vi "Execute VI Analyzer Tests.vi"(8 "error in":errorcluster, 9 "File Name":string, 10 "File List":path[](array[path]), 11 "Peer Review in":refnum<class "Peer Review.lvclass">) -> (0 "error out":errorcluster, 3 "Peer Review out":refnum<class "Peer Review.lvclass">)   [LabVIEW 2020, in "Peer Review.lvclass"]
uses:
  Peer Review.lvclass
  Peer Review.lvclass/Peer Review.ctl
  <vilib>/addons/analyzer/NI_VIAnalyzerTKVIs.lvlib
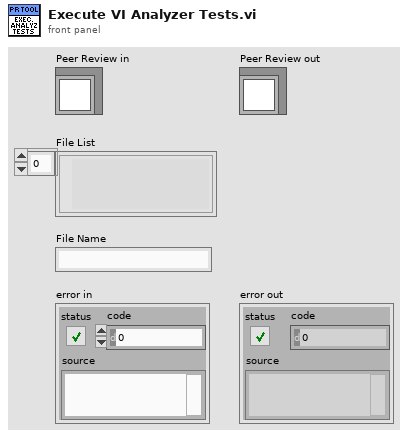
[diagram p1: front panel]
types:
  T1 = typedef "Peer Review.lvclass/File Info.ctl" = cluster{"File ID":i32, "Commit ID":i32, "Reviewed Hash":string, "Relative Path":string, "File Path":path, "File Checksum":string, "State":T2, "FP Changes":i32, "BD Changes":i32, "FP Bounds Error":dbl, "BD Bounds Error":dbl, "Lines Added":i32, "Lines Removed":i32, "Analysis Passes":i32, "Analysis Fails":i32, "Attribute Changes":i32, "Reentrancy State":string, "Cyclomatic Complexity":i32, "Node Count":i32, "Revision Number":u32, "LabVIEW Version":string, "Description":string, "Master Path":path, "Master Checksum":string, "VI Type":T3, "LabVIEW File":bool, "Review Complete":bool, "File Ref":refnum<vi>}
  T2 = typedef "Peer Review.lvclass/File State.ctl" = enum16{"Interrogation Needed", "Modified", "Deleted", "Added", "Matches Previous", "No Changes", "Moved"}
  T3 = typedef "Peer Review.lvclass/VI Type.ctl" = enum32{"invalid VI type", "Standard VI", "Control VI", "Global VI", "Polymorphic VI", "Configuration VI", "SubSystem", "Facade VI", "Method VI", "Statechart Diagram VI"}
  T4 = typedef "VIAnAPI Ref.ctl" = refnum<k1>
  T5 = typedef "VIAnCtl Results.ctl" = cluster{"Test Name":string, "Results Data":T6[], "Status":T7, "Exceed Max Fails?":bool}
  T6 = typedef "VIAnCtl ResultsData (index).ctl" = cluster{"Result Message":string, "Ref Index":i32}
  T7 = typedef "VIAnCtl ResultStatus.ctl" = enum16{"Pass", "Fail", "Skipped", "VI not loadable", "Test not loadable", "Test not runnable", "Test error out"}
  T8 = typedef "VIAnRes Parsed Results Data (by VI).ctl" = cluster{"VI Path":path, "Pass":cluster{"row":i32, "column":i32}[], "Fail":cluster{"row":i32, "column":i32}[], "Skipped":cluster{"row":i32, "column":i32}[], "VI not loadable":cluster{"row":i32, "column":i32}[], "Test not loadable":cluster{"row":i32, "column":i32}[], "Test not runnable":cluster{"row":i32, "column":i32}[], "Test error out":cluster{"row":i32, "column":i32}[]}
  T9 = typedef "VIAnRes Parsed Results Data (by Test).ctl" = cluster{"Test Name":string, "Pass":cluster{"VI Path":path, "index":cluster{"row":i32, "column":i32}}[], "Fail":cluster{"VI Path":path, "index":cluster{"row":i32, "column":i32}}[], "Skipped":cluster{"VI Path":path, "index":cluster{"row":i32, "column":i32}}[]}
  T10 = typedef "VIAnCtl Test Config Data.ctl" = cluster{"Test Name":string, "Config Ref":refnum<vi>, "Ref Valid?":bool, "Test Ranking":T11, "Max Failures":u32, "Test Path":path, "Control Values":T12[], "Selected?":bool}
  T11 = typedef "VIAnCtl TestRanking.ctl" = u16
  T12 = typedef "VIAnCtl Config Control Value.ctl" = cluster{"Control Name":string, "Control Value":variant}
  T13 = cluster{"Raw Results":T5[][], "Parsed Results Data (by VI)":T8[], "Parsed Results Data (by Test)":T9[], "Summary Statistics":cluster{"Passed Tests":i32, "Failed Tests":i32, "Skipped Tests":i32, "VIs not loadable":i32, "Tests not loadable":i32, "Tests not runnable":i32, "Test error out":i32, "Start Time":u32, "Total Time (s)":dbl}, "Test Config Data":T10[]}
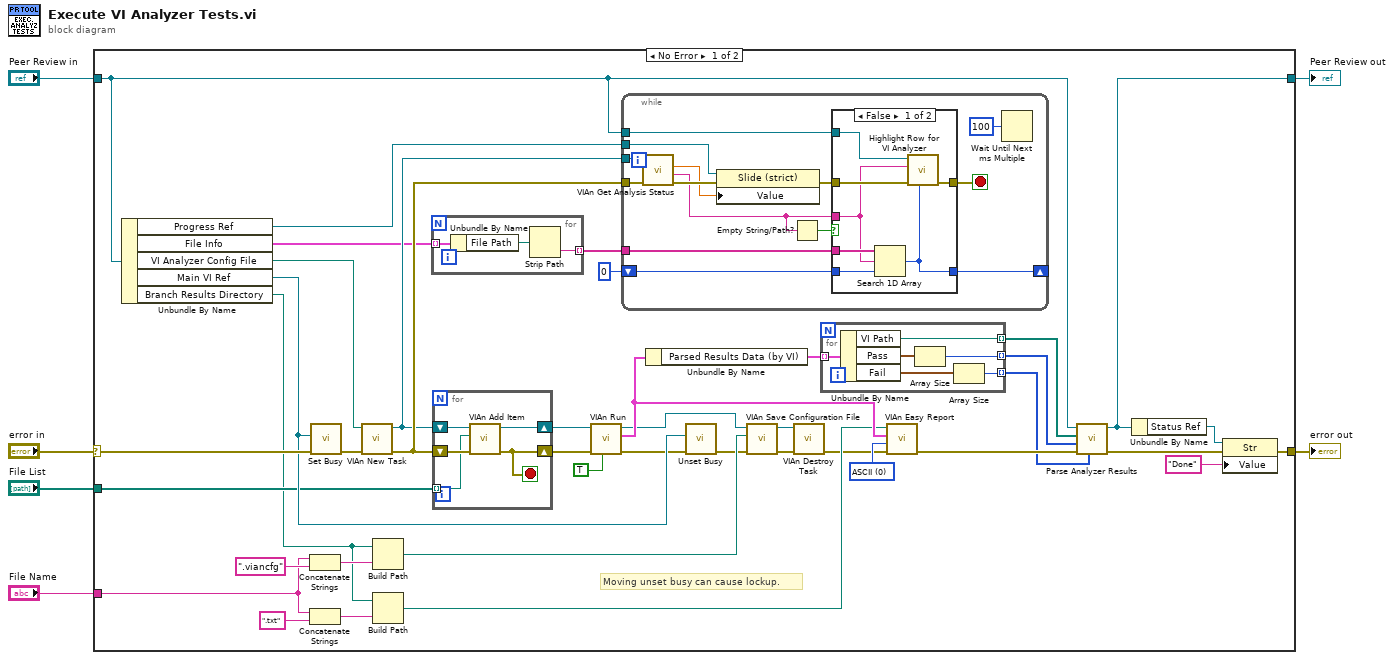
[diagram p0: block diagram]
diagram:
  n1 = case shown="No Error" "error in" {
    selector: "error in" -> [w33 w86]
    tunnel: [w13 w86] -> w6
    tunnel: "Peer Review in" -> [w15 w85]
    tunnel: [w14 w85] -> w4
    tunnel: "File Name" -> [w11 _]
    tunnel: "File List" -> [w26 _]
    frame No Error {
      w22 = u16 0 items=["ASCII", "HTML", "RSL File"] ("Report Save Type (ASCII)")
      # "Moving unset busy can cause lockup."
      n2 = Unbundle By Name(w15) -> ("Progress Ref"=w7:refnum<vi>, "File Info"=w10:T1[], "VI Analyzer Config File"=w47:path, "Main VI Ref"=w31:refnum<vi>, "Branch Results Directory"=w16:path)
      n3 = Concatenate Strings(w11, ".viancfg") -> (w35:string)
      n4 = Concatenate Strings(w11, ".txt") -> (w36:string)
      n5 = call <vilib>:"Set Busy.vi"("error in (no error)"=w33, "VI reference (current VI)"=w31) -> ("error out"=w18:errorcluster)  [unwired: 8 in, 1 out]
      n6 = call <vilib>:"VIAn New Task.vi"("error in (no error)"=w18, "Path to Configuration File"=w47) -> ("error out"=w20:errorcluster, "VI Analyzer Task"=w19:T4)  [unwired: 1 in, 7 out]
      n7 = Build Path(base path=w16, name or relative path=w35) -> (appended path=w37:path)
      n8 = Build Path(base path=w16, name or relative path=w36) -> (appended path=w38:path)
      n9 = for {
        tunnel: w10 -> [w50] mode=indexing
        tunnel: [w48] -> w8 mode=indexing
        n10 = Unbundle By Name(w50) -> ("File Path"=w49:path)
        n11 = Strip Path(path=w49) -> (name=w48:string)  [unwired: 1 out]
      }
      n12 = for {
        shift-right: [w80] -> w23
        shift-left: w20 -> [w84]
        shift-right: [w83] -> w24
        shift-left: w19 -> [w82]
        tunnel: w26 -> [w81] mode=indexing
        stop <- w80 stop-if-true
        n13 = call <vilib>:"VIAn Add Item.vi"("error in (no error)"=w84, "Item to Add"=w81, "VI Analyzer Task in"=w82) -> ("error out"=w80:errorcluster, "VI Analyzer Task out"=w83:T4)  [unwired: 7 in]
      }
      n14 = call <vilib>:"VIAn Run.vi"("Show Results Window?"=TRUE, "error in (no error)"=w23, "VI Analyzer Task in"=w24) -> ("error out"=w25:errorcluster, "Analysis Results"=w40:T13, "VI Analyzer Task out"=w27:T4)  [unwired: 6 out]
      n15 = while {
        tunnel: w19 -> [w70]
        tunnel: w20 -> [w69]
        tunnel: w15 -> [w66]
        shift-right: [w63] -> _
        shift-left: 0 -> [w64]
        tunnel: w8 -> [w65]
        tunnel: w7 -> [w58]
        stop <- w67 stop-if-true
        n16 = call <vilib>:"VIAn Get Analysis Status.vi"("error in (no error)"=w69, "VI Analyzer Task in"=w70) -> ("error out"=w61:errorcluster, "VI in Analysis"=w57:string, "Percent Complete"=w59:dbl)  [unwired: 7 out]
        n17 = property class="Slide (strict)"(reference=w58, error in=w61, "Value"=w59) -> (error out=w60:errorcluster)  [unwired: 1 out]
        n18 = Empty String/Path?(string/path=w57) -> (empty?=w62:bool)
        n19 = case shown="False" w62 {
          tunnel: w60 -> [w77 w79]
          tunnel: [w76 w79] -> w67
          tunnel: w66 -> [w75 _]
          tunnel: w65 -> [w74 _]
          tunnel: w64 -> [w73 w78]
          tunnel: [w72 w78] -> w63
          tunnel: w57 -> [w71 _]
          frame False {
            n20 = Search 1D Array(1D array=w74, element=w71, start index (0)=w73) -> (index of element=w72:i32)
            n21 = call "Highlight Row for VI Analyzer.vi"("File Index"=w72, "error in"=w77, "Review File"=w71, "Peer Review"=w75) -> ("error out"=w76:errorcluster)  [unwired: 7 in]
          }
          frame True {
          }
        }
        n22 = Wait Until Next ms Multiple(millisecond multiple=u32 100 ("milliseconds to wait")) -> ()  [unwired: 1 out]
      }
      n23 = Unbundle By Name(w40) -> ("Parsed Results Data (by VI)"=w41:T8[])
      n24 = call <vilib>:"Unset Busy.vi"("error in (no error)"=w25, "VI reference (current VI)"=w31) -> ("error out"=w29:errorcluster)  [unwired: 9 out]
      n25 = call <vilib>:"VIAn Save Configuration File.vi"("error in (no error)"=w29, "Path to Configuration File"=w37, "VI Analyzer Task in"=w27) -> ("error out"=w30:errorcluster, "VI Analyzer Task out"=w28:T4)  [unwired: 7 in]
      n26 = call <vilib>:"VIAn Destroy Task.vi"("error in (no error)"=w30, "VI Analyzer Task in"=w28) -> ("error out"=w21:errorcluster)  [unwired: 9 out]
      n27 = for {
        tunnel: w41 -> [w56] mode=indexing
        tunnel: [w53] -> w42 mode=indexing
        tunnel: [w52] -> w43 mode=indexing
        tunnel: [w51] -> w44 mode=indexing
        n28 = Unbundle By Name(w56) -> ("VI Path"=w53:path, "Pass"=w55:cluster{"row":i32, "column":i32}[], "Fail"=w54:cluster{"row":i32, "column":i32}[])
        n29 = Array Size(array=w55) -> (size(s)=w52:i32)
        n30 = Array Size(array=w54) -> (size(s)=w51:i32)
      }
      n31 = call <vilib>:"VIAn Easy Report.vi"("error in (no error)"=w21, "Report Save Type (ASCII)"=w22, "Analysis Results"=w40, "Report Save Path"=w38) -> ("error out"=w46:errorcluster)  [unwired: 3 in, 4 out]
      n32 = call "Parse Analyzer Results.vi"("Fails"=w44, "error in"=w46, "Passes"=w43, "VI Paths"=w42, "Peer Review in"=w15) -> ("error out"=w45:errorcluster, "Peer Review out"=w14:refnum<class "Peer Review.lvclass">)  [unwired: 5 in]
      n33 = Unbundle By Name(w14) -> ("Status Ref"=w12:refnum<vi>)
      n34 = property on="Property Node" class="Str"(reference=w12, error in=w45, "Value"="Done") -> (error out=w13:errorcluster)  [unwired: 1 out]
    }
    frame Error {
    }
  }
  "error out" <- w6
  "Peer Review out" <- w4
